vi "Main - Submodules Init.vi"(7 "Kill if running?":bool, 8 "Error In":errorcluster, 10 "VIs name":string[](array[string]), 11 "Path to Modules Folder":path) -> (0 "Error Out":errorcluster, 3 "Module Refnum":refnum<vi>[](array[refnum]))   [LabVIEW 2020]
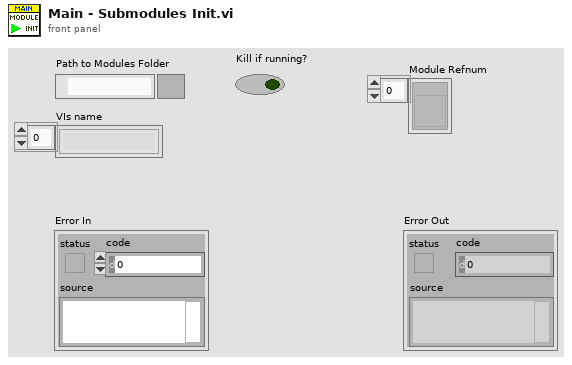
[diagram p1: front panel]
types:
  T1 = enum32{"Bad", "Idle", "Run top level", "Running"}
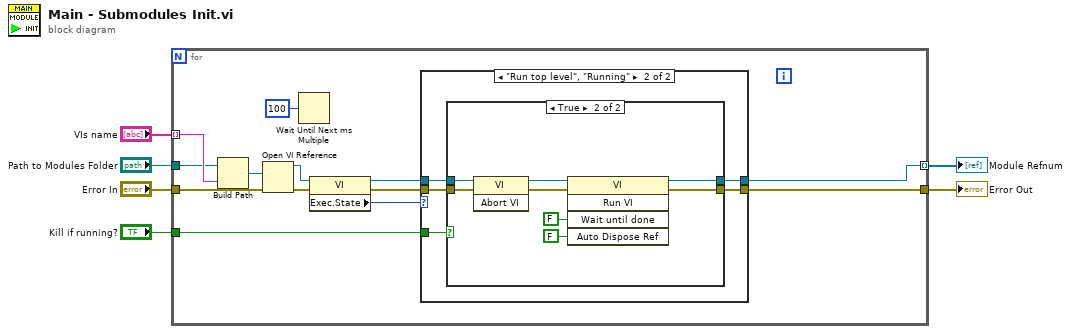
[diagram p0: block diagram]
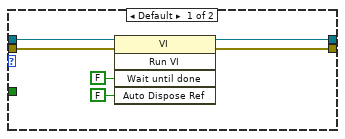
[diagram p2: hidden frame]
diagram:
  n1 = for {
    tunnel: "Error In" -> [w19]
    tunnel: [w16] -> w6
    tunnel: [w7] -> w4 mode=indexing
    tunnel: "VIs name" -> [w12] mode=indexing
    tunnel: "Path to Modules Folder" -> [w11]
    tunnel: "Kill if running?" -> [w9]
    n2 = Build Path(base path=w11, name or relative path=w12) -> (appended path=w10:path)
    n3 = Open VI Reference(vi path=w10, error in (no error)=w19) -> (vi reference=w15:refnum<vi>, error out=w18:errorcluster)  [unwired: 4 in]
    n4 = Wait Until Next ms Multiple(millisecond multiple=u32 100) -> ()  [unwired: 1 out]
    n5 = property class="VI"(reference=w15, error in=w18) -> (reference out=w13:refnum<vi>, error out=w17:errorcluster, "Exec.State"=w14:T1)
    n6 = case shown="\"Run top level\", \"Running\"" w14 {
      tunnel: w17 -> [w25 w30]
      tunnel: w13 -> [w21 w28]
      tunnel: [w20 w27] -> w7
      tunnel: [w24 w29] -> w16
      tunnel: w9 -> [_ w26]
      frame Default {
        n7 = invoke class="VI" method="Run VI"(reference=w21, error in=w25, "Wait until done"=FALSE ("Wait Until Done"), "Auto Dispose Ref"=FALSE ("Auto Dispose Reference")) -> (reference out=w20:refnum<vi>, error out=w24:errorcluster)  [unwired: 1 in, 3 out]
      }
      frame "Run top level", "Running" {
        n8 = case shown="True" w26 {
          tunnel: w30 -> [w32 w40]
          tunnel: w28 -> [w31 w37]
          tunnel: [w31 w33] -> w27
          tunnel: [w32 w38] -> w29
          frame False {
          }
          frame True {
            n9 = invoke class="VI" method="Abort VI"(reference=w37, error in=w40) -> (reference out=w34:refnum<vi>, error out=w39:errorcluster)  [unwired: 1 in, 1 out]
            n10 = invoke class="VI" method="Run VI"(reference=w34, error in=w39, "Wait until done"=FALSE ("Wait Until Done"), "Auto Dispose Ref"=FALSE ("Auto Dispose Reference")) -> (reference out=w33:refnum<vi>, error out=w38:errorcluster)  [unwired: 1 in, 3 out]
          }
        }
      }
    }
  }
  "Error Out" <- w6
  "Module Refnum" <- w4
